vi "ATE_Plate_SafeState_TxDisable.vi"(2 "error in (no error)":errorcluster) -> (0 "error out":errorcluster)   [LabVIEW 2009]
doc: "Set the ATE plate switches in safe state leave Tx DISABLED. We do not move any WG switches.\nDo not enable Tx afterwards."
panel:
  # "Set the ATE plate switches in safe state and leave Tx disabled.  DO not move the WG switches.\nOvertly disable Tx, although UltraSafe disables Tx upon entry. Leave Tx DISABLED."
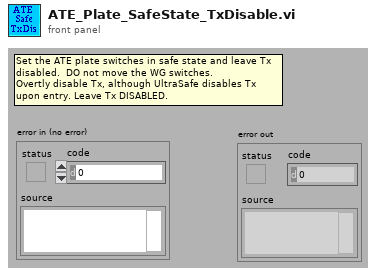
[diagram p1: front panel]
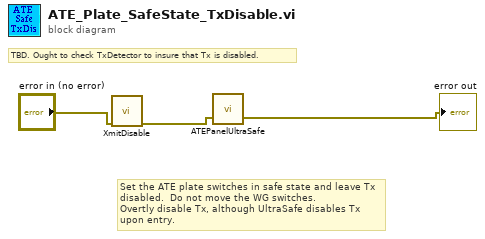
[diagram p0: block diagram]
diagram:
  # "TBD. Ought to check TxDetector to insure that Tx is disabled."
  # "Set the ATE plate switches in safe state and leave Tx disabled.  Do not move the WG switches.\nOvertly disable Tx, although UltraSafe disables Tx upon entry."
  n1 = call "XmitDisable.vi"("error in (no error)"="error in (no error)") -> ("error out"=w2:errorcluster)  [unwired: 1 in, 5 out]
  n2 = call "ATEPanelUltraSafe.vi"("error in (no error)"=w2) -> ("Error out"=→"error out":errorcluster)  [unwired: 2 in]
